vi "Unsubscribe (Enqueuer and Msg).vi"(8 "error in":errorcluster, 9 "Message":refnum<class "Message.lvclass">, 10 "Enqueuer":refnum<class "Message Enqueuer.lvclass">, 11 "MVC Subscription in":refnum<class "MVC Subscription.lvclass">) -> (0 "error out":errorcluster, 3 "MVC Subscription out":refnum<class "MVC Subscription.lvclass">)   [LabVIEW 2016, in "MVC Subscription.lvlib" / "MVC Subscription.lvclass"]
uses:
  MVC Subscription.lvclass
  <vilib>/ActorFramework/Message Enqueuer/Message Enqueuer.lvclass
  <vilib>/ActorFramework/Message/Message.lvclass
  Cluster - Individual Subscription.ctl
  MVC Subscription.lvclass/MVC Subscription.ctl
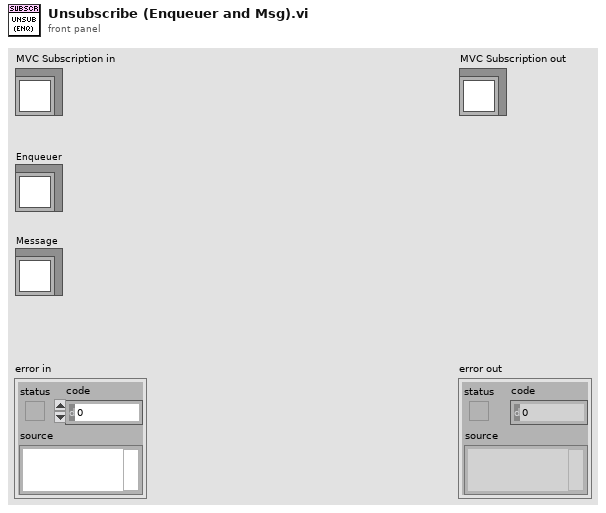
[diagram p1: front panel]
types:
  T1 = typedef "MVC Subscription.lvlib/MVC Subscription.lvclass/Cluster - Individual Subscription.ctl" = cluster{"Enqueuer":refnum<class "Message Enqueuer.lvclass">, "Message":refnum<class "Message.lvclass">}
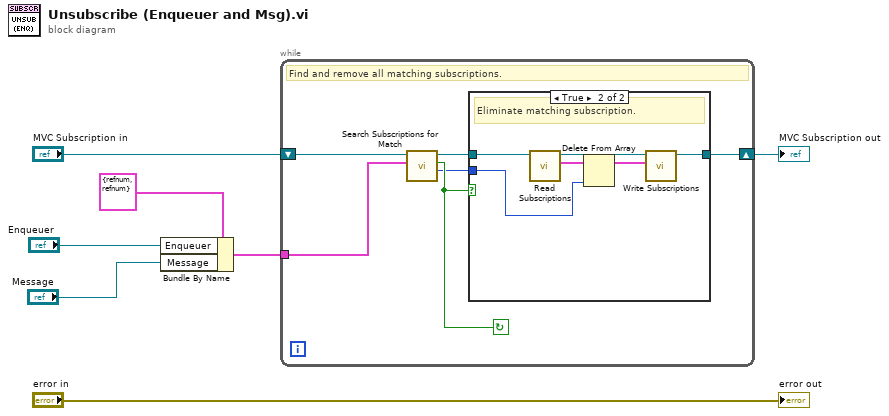
[diagram p0: block diagram]
diagram:
  n1 = Bundle By Name(cluster=T1 {"Enqueuer"=refnum, "Message"=refnum} ("Subscription"), "Enqueuer"="Enqueuer", "Message"="Message") -> (w3:T1)
  n2 = while {
    tunnel: w3 -> [w12]
    shift-right: [w9] -> w5
    shift-left: "MVC Subscription in" -> [w13]
    stop <- w11 continue-if-true
    # "Find and remove all matching subscriptions."
    n3 = call "Search Subscriptions for Match.vi"("Subscription"=w12, "MVC Subscription in"=w13) -> ("Index"=w10:i32, "Found"=w11:bool, "MVC Subscription out"=w8:refnum<class "MVC Subscription.lvclass">)  [unwired: 7 in]
    n4 = case shown="True" w11 {
      tunnel: w10 -> [_ w15]
      tunnel: [w14 w18] -> w9
      tunnel: w8 -> [w14 w20]
      frame False {
      }
      frame True {
        # "Eliminate matching subscription."
        n5 = call "Read Subscriptions.vi"("MVC Subscription in"=w20) -> ("Subscriptions"=w17:T1[], "MVC Subscription out"=w19:refnum<class "MVC Subscription.lvclass">)  [unwired: 9 in]
        n6 = Delete From Array(array=w17, index=w15) -> (array with subset deleted=w16:T1[])  [unwired: 1 in, 1 out]
        n7 = call "Write Subscriptions.vi"("Subscriptions"=w16, "MVC Subscription in"=w19) -> ("MVC Subscription out"=w18:refnum<class "MVC Subscription.lvclass">)  [unwired: 9 in]
      }
    }
  }
  "MVC Subscription out" <- w5
  "error out" <- "error in"
